vi "GraphAttribute.vi"() -> ()   [LabVIEW 2012, in "WaveGraphX.xctl"]
uses:
  WaveGraphX.xctl
  <resource>/importtools/Common/Event/NISAST Event.lvclass
  GraphStates.ctl
panel:
  in  "曲线条数":u8
  in  "AttrCluster":T1={"曲线条数"=3, "曲线属性簇数组"=[{"曲线_曲线"=0, "曲线_颜色"=16711717, "曲线_线条样式"=0, "曲线_线条宽度"=0, "曲线_直方图"=0, "曲线_插值"=0, "曲线_填充基线"=0, "曲线_点样式"=0}, {"曲线_曲线"=1, "曲线_颜色"=786687, "曲线_线条样式"=1, "曲线_线条宽度"=0, "曲线_直方图"=0, "曲线_插值"=0, "曲线_填充基线"=0, "曲线_点样式"=0}, {"曲线_曲线"=2, "曲线_颜色"=56357, "曲线_线条样式"=2, "曲线_线条宽度"=0, "曲线_直方图"=0, "曲线_插值"=0, "曲线_填充基线"=0, "曲线_点样式"=0}], "文本属性簇数组"=[{"文本_文本"=0, "文本"="标题", "字体"=0, "颜色"=0, "大小"=0, "加粗"=TRUE, "斜体"=FALSE, "下划线"=FALSE}, {"文本_文本"=1, "文本"="", "字体"=0, "颜色"=0, "大小"=0, "加粗"=FALSE, "斜体"=TRUE, "下划线"=FALSE}, {"文本_文本"=2, "文本"="", "字体"=0, "颜色"=0, "大小"=0, "加粗"=FALSE, "斜体"=FALSE, "下划线"=TRUE}, {"文本_文本"=3, "文本"="", "字体"=0, "颜色"=0, "大小"=0, "加粗"=TRUE, "斜体"=TRUE, "下划线"=TRUE}], "信息属性簇"={"图例"=TRUE, "信息_统计量"=FALSE, "信息_统计量_有效值"=TRUE, "信息_统计量_最大值"=TRUE, "信息_统计量_最小值"=FALSE, "信息_统计量_峰峰值"=FALSE, "信息_统计量_均值"=FALSE, "信息_统计量_方差"=FALSE, "信息_统计量_所有通道"=FALSE, "光标列表"=1, "数量"=1.0, "排列"=0, "格式"=0, "精度"=3.0}} {"信息属性簇"."格式" items=["十进制", "科学值"]; "信息属性簇"."排列" items=["幅值"]; "信息属性簇"."光标列表" items=["单光标", "双光标", "峰值光标"]; "曲线属性簇数组"."曲线_填充基线" items=["无", "零", "负无穷大", "正无穷大"]; "曲线属性簇数组"."曲线_线条宽度" items=["0", "1", "2", "3", "4", "5"]; "曲线属性簇数组"."曲线_线条样式" items=["实线", "粗虚线", "细虚线", "点划线", "双点划线"]}
  in  "Event In":refnum<class "NISAST Event.lvclass">
  in  "应用":bool
  in  "取消":bool
  in  "确定":bool
  in  "选项卡控件":enum32{"曲线", "文本", "信息"}(tab)
  in  "曲线_曲线":i32(listbox) caption="曲线"
  in  "曲线_颜色":u32(colorbox) caption="颜色"
  in  "曲线_线条宽度":u16(ring) caption="线条宽度" items=["0", "1", "2", "3", "4", "5"]
  in  "曲线_线条样式":u16(ring) caption="线条样式" items=["实线", "粗虚线", "细虚线", "点划线", "双点划线"]
  in  "曲线_直方图":u16(ring) caption="直方图"
  in  "曲线_插值":u16(ring) caption="插值"
  in  "曲线_填充基线":u16(ring) caption="填充基线" items=["无", "零", "负无穷大", "正无穷大"]
  in  "曲线_点样式":u16(ring) caption="点样式"
  in  "加粗":bool
  in  "大小":u16(ring)
  in  "文本":string
  in  "文本_文本":i32(listbox) caption="文本"
  in  "字体":u16(ring)
  in  "颜色":u16(ring)
  in  "斜体":bool
  in  "下划线":bool
  in  "格式":u16(ring) items=["十进制", "科学值"]
  in  "信息_统计量_所有通道":bool
  in  "信息_统计量":bool
  in  "图例":bool
  in  "信息_统计量_有效值":bool
  in  "信息_统计量_最大值":bool
  in  "信息_统计量_最小值":bool
  in  "信息_统计量_峰峰值":bool
  in  "信息_统计量_均值":bool
  in  "信息_统计量_方差":bool
  in  "光标列表":u16(ring) items=["单光标", "双光标", "峰值光标"]
  in  "数量":dbl=1.0
  in  "排列":u16(ring) items=["幅值"]
  in  "精度":dbl=3.0
  # "光标"
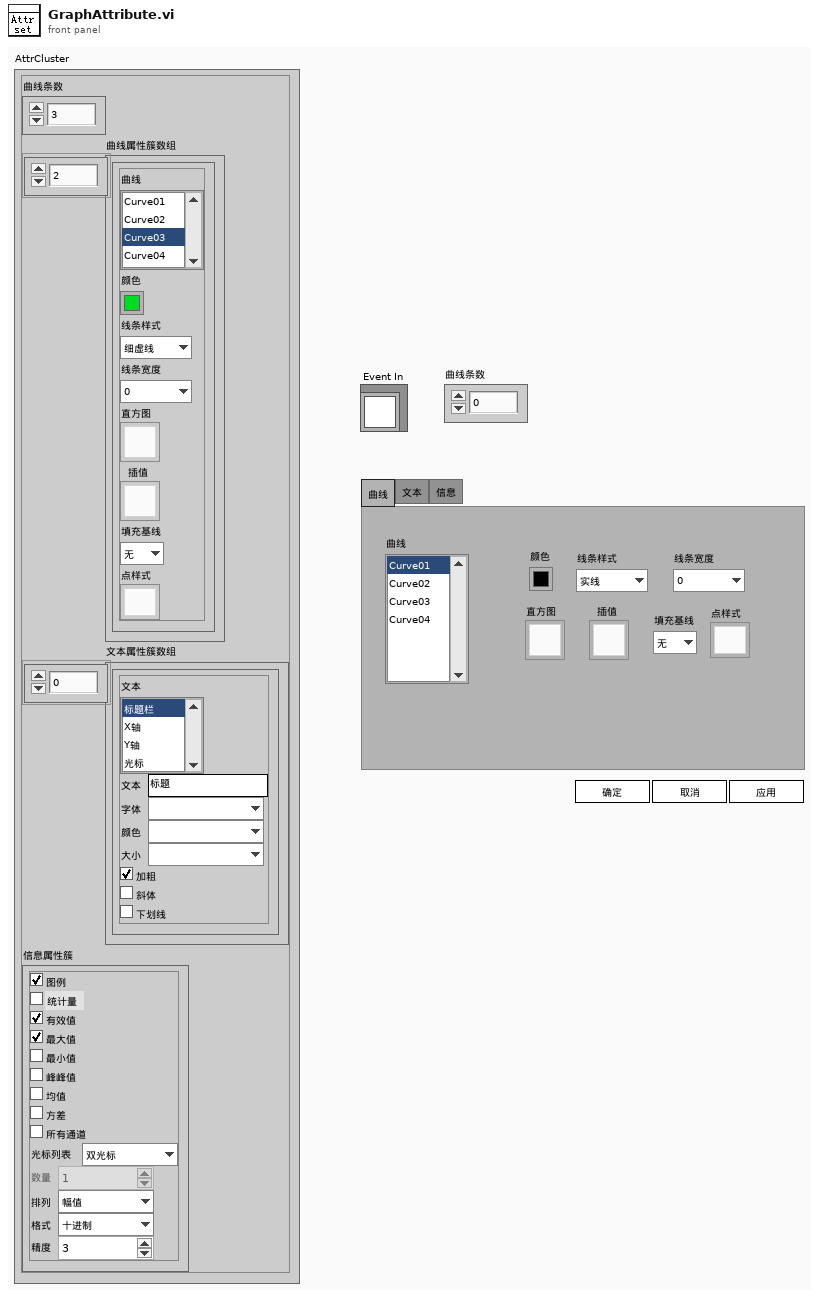
[diagram p1: front panel]
types:
  T1 = typedef "WaveGraphX.xctl/GraphStates.ctl" = cluster{"曲线条数":u8, "曲线属性簇数组":cluster{"曲线_曲线":i32, "曲线_颜色":u32, "曲线_线条样式":u16, "曲线_线条宽度":u16, "曲线_直方图":u16, "曲线_插值":u16, "曲线_填充基线":u16, "曲线_点样式":u16}[], "文本属性簇数组":cluster{"文本_文本":i32, "文本":string, "字体":u16, "颜色":u16, "大小":u16, "加粗":bool, "斜体":bool, "下划线":bool}[], "信息属性簇":cluster{"图例":bool, "信息_统计量":bool, "信息_统计量_有效值":bool, "信息_统计量_最大值":bool, "信息_统计量_最小值":bool, "信息_统计量_峰峰值":bool, "信息_统计量_均值":bool, "信息_统计量_方差":bool, "信息_统计量_所有通道":bool, "光标列表":u16, "数量":dbl, "排列":u16, "格式":u16, "精度":dbl}}
  T2 = cluster{"曲线_曲线":i32, "曲线_颜色":u32, "曲线_线条样式":u16, "曲线_线条宽度":u16, "曲线_直方图":u16, "曲线_插值":u16, "曲线_填充基线":u16, "曲线_点样式":u16}[]
  T3 = cluster{"文本_文本":i32, "文本":string, "字体":u16, "颜色":u16, "大小":u16, "加粗":bool, "斜体":bool, "下划线":bool}[]
  T4 = cluster{"图例":bool, "信息_统计量":bool, "信息_统计量_有效值":bool, "信息_统计量_最大值":bool, "信息_统计量_最小值":bool, "信息_统计量_峰峰值":bool, "信息_统计量_均值":bool, "信息_统计量_方差":bool, "信息_统计量_所有通道":bool, "光标列表":u16, "数量":dbl, "排列":u16, "格式":u16, "精度":dbl}
  T5 = cluster{"曲线_曲线":i32, "曲线_颜色":u32, "曲线_线条样式":u16, "曲线_线条宽度":u16, "曲线_直方图":u16, "曲线_插值":u16, "曲线_填充基线":u16, "曲线_点样式":u16}
  T6 = cluster{"文本_文本":i32, "文本":string, "字体":u16, "颜色":u16, "大小":u16, "加粗":bool, "斜体":bool, "下划线":bool}
  T7 = enum8{"Enabled", "Disabled", "Disabled and Grayed Out"}
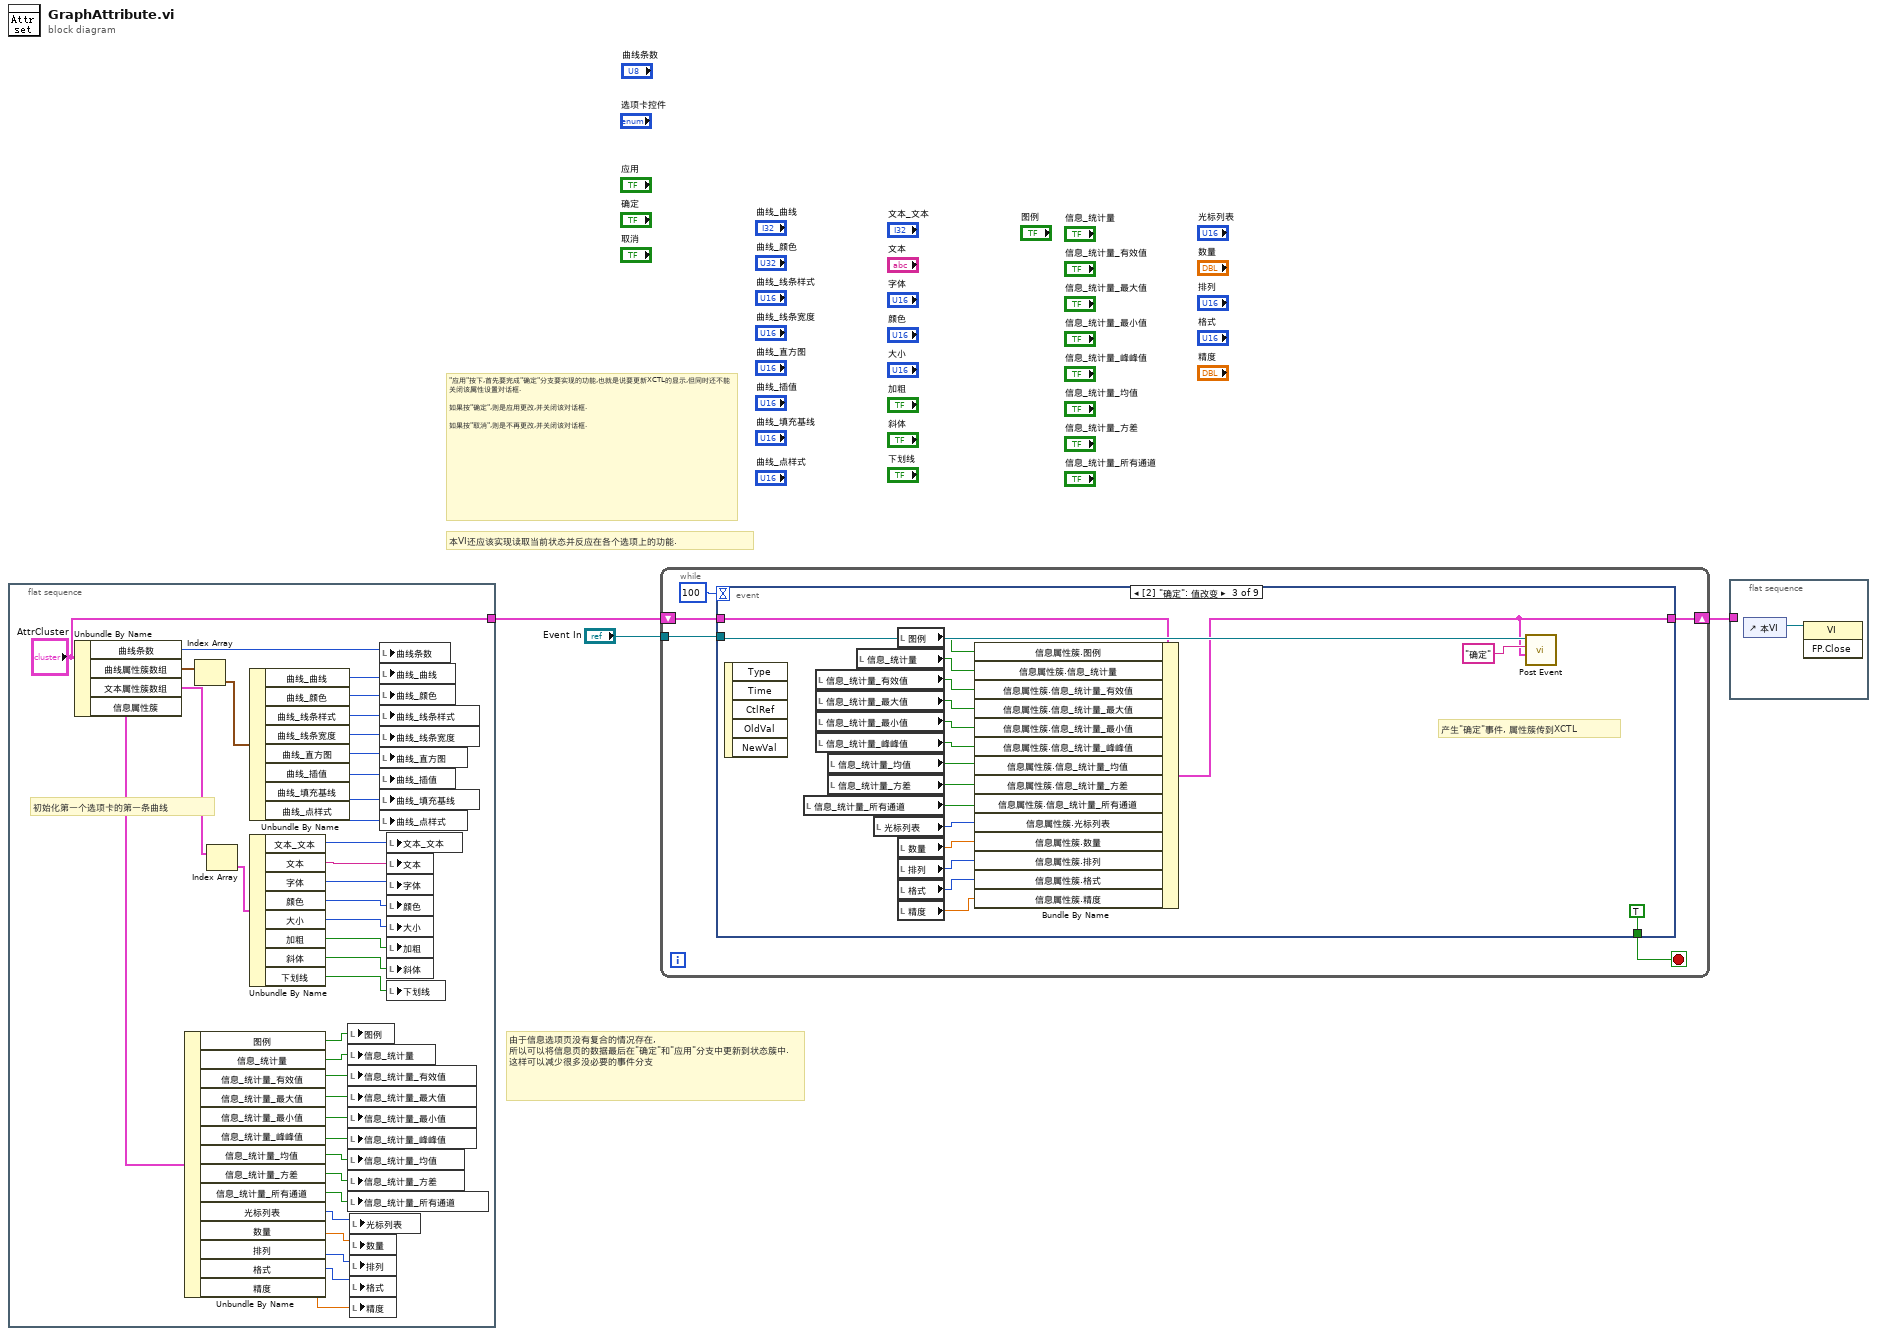
[diagram p0: block diagram]
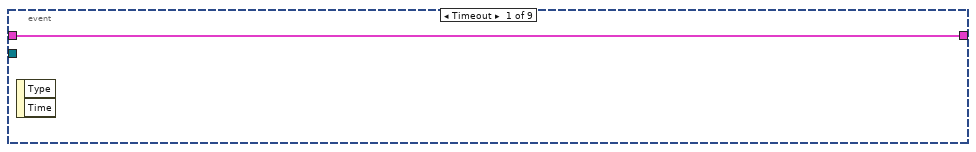
[diagram p2: hidden frame]
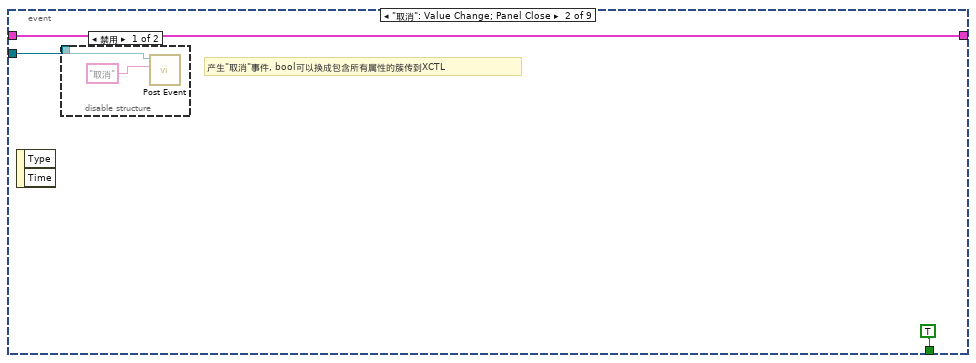
[diagram p3: hidden frame]
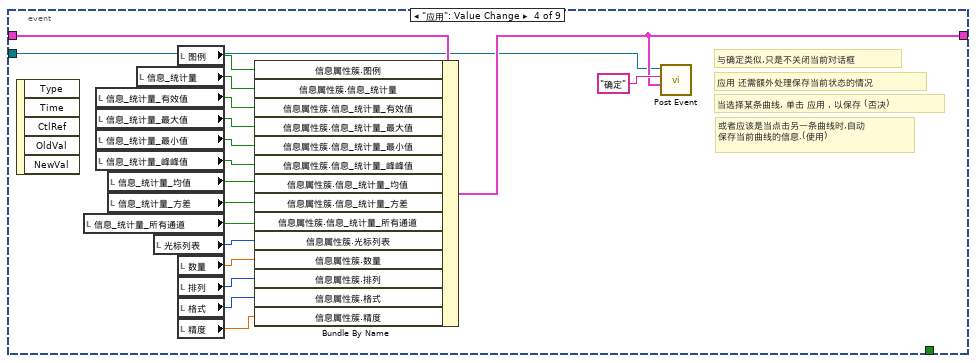
[diagram p5: hidden frame]
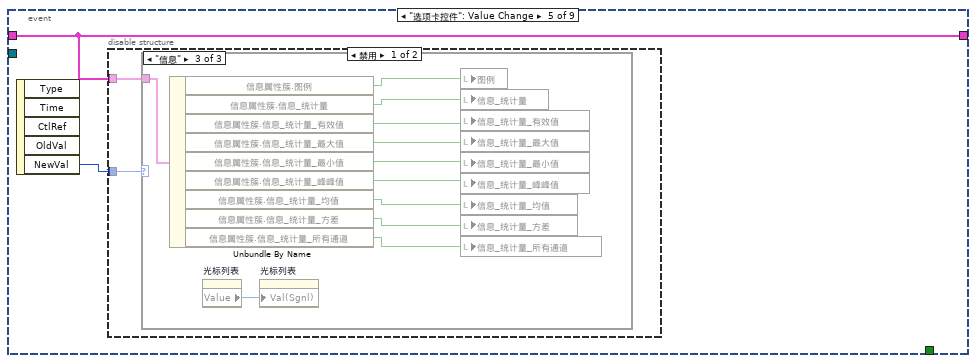
[diagram p6: hidden frame]
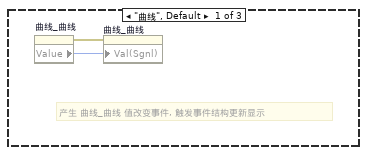
[diagram p7: hidden frame]
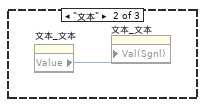
[diagram p8: hidden frame]
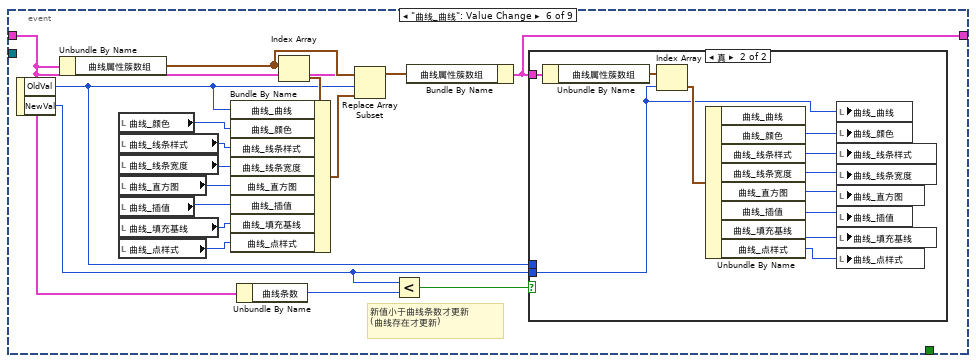
[diagram p10: hidden frame]
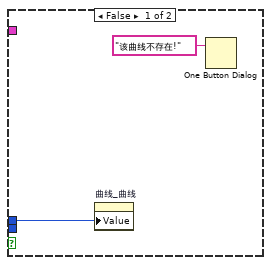
[diagram p11: hidden frame]
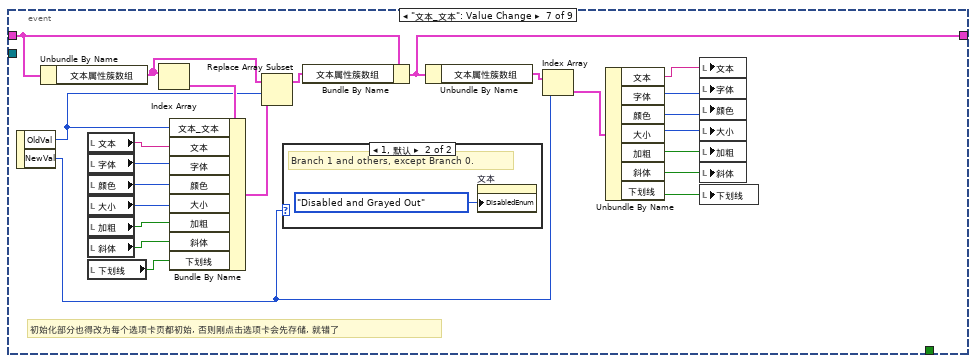
[diagram p12: hidden frame]
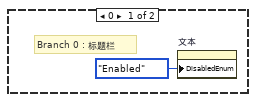
[diagram p13: hidden frame]
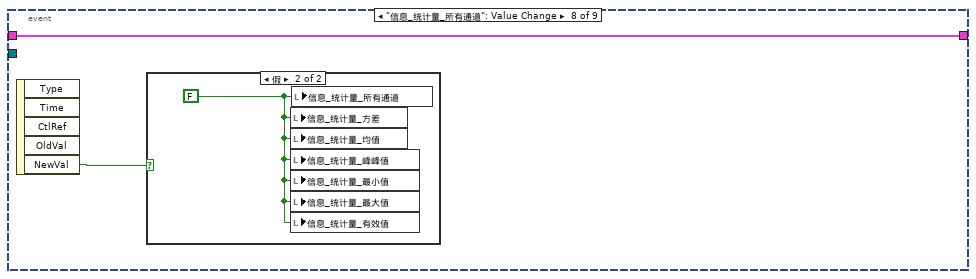
[diagram p14: hidden frame]
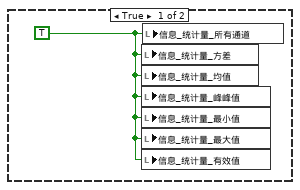
[diagram p15: hidden frame]
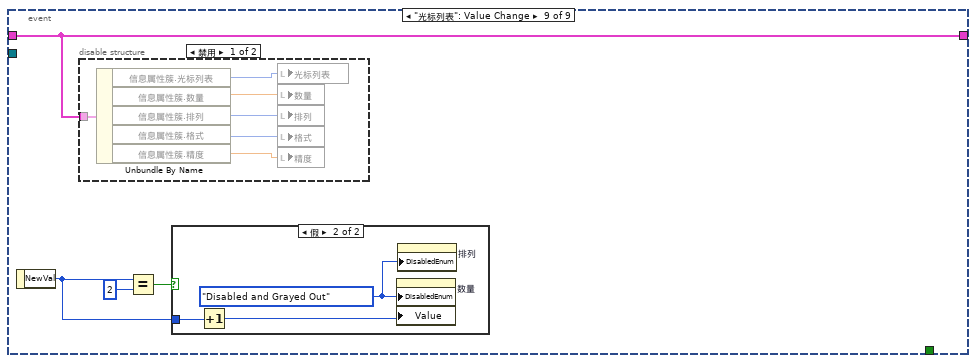
[diagram p16: hidden frame]
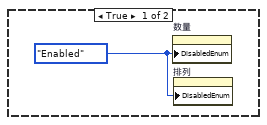
[diagram p18: hidden frame]
diagram:
  # "由于信息选项页没有复合的情况存在, 所以可以将信息页的数据最后在\"确定\"和\"应用\"分支中更新到状态簇中.这样可以减少很多没必要的事件分支"
  # "本VI还应该实现读取当前状态并反应在各个选项上的功能."
  # "\"应用\"按下,首先要完成\"确定\"分支要实现的功能,也就是说要更新XCTL的显示,但同时还不能关闭该属性设置对话框.\n\n如果按\"确定\",则是应用更改,并关闭该对话框.\n\n如果按\"取消\",则是不再更改,并关闭该对话框."
  n1 = flat-sequence {
    tunnel: ["AttrCluster"] -> w2
    frame #0 {
      # "初始化第一个选项卡的第一条曲线"
      n2 = Unbundle By Name("AttrCluster") -> ("曲线条数"=w40:u8, "曲线属性簇数组"=w39:T2, "文本属性簇数组"=w28:T3, "信息属性簇"=w18:T4)
      n3 = Unbundle By Name(w18) -> ("图例"=w10:bool, "信息_统计量"=w9:bool, "信息_统计量_有效值"=w17:bool, "信息_统计量_最大值"=w16:bool, "信息_统计量_最小值"=w15:bool, "信息_统计量_峰峰值"=w14:bool, "信息_统计量_均值"=w13:bool, "信息_统计量_方差"=w12:bool, "信息_统计量_所有通道"=w11:bool, "光标列表"=w8:u16, "数量"=w7:dbl, "排列"=w6:u16, "格式"=w5:u16, "精度"=w4:dbl)
      n4 = Index Array(array=w39) -> (element=w38:T5)  [unwired: 1 in]
      n5 = Index Array(array=w28) -> (element=w27:T6)  [unwired: 1 in]
      n6 = Unbundle By Name(w38) -> ("曲线_曲线"=w37:i32, "曲线_颜色"=w36:u32, "曲线_线条样式"=w35:u16, "曲线_线条宽度"=w34:u16, "曲线_直方图"=w33:u16, "曲线_插值"=w32:u16, "曲线_填充基线"=w31:u16, "曲线_点样式"=w30:u16)
      n7 = Unbundle By Name(w27) -> ("文本_文本"=w19:i32, "文本"=w26:string, "字体"=w25:u16, "颜色"=w24:u16, "大小"=w23:u16, "加粗"=w22:bool, "斜体"=w21:bool, "下划线"=w20:bool)
      n8 = local write "图例"(w10) -> ()
      n9 = local write "信息_统计量"(w9) -> ()
      n10 = local write "信息_统计量_有效值"(w17) -> ()
      n11 = local write "信息_统计量_最大值"(w16) -> ()
      n12 = local write "信息_统计量_最小值"(w15) -> ()
      n13 = local write "信息_统计量_峰峰值"(w14) -> ()
      n14 = local write "信息_统计量_均值"(w13) -> ()
      n15 = local write "信息_统计量_方差"(w12) -> ()
      n16 = local write "信息_统计量_所有通道"(w11) -> ()
      n17 = local write "光标列表"(w8) -> ()
      n18 = local write "数量"(w7) -> ()
      n19 = local write "排列"(w6) -> ()
      n20 = local write "格式"(w5) -> ()
      n21 = local write "精度"(w4) -> ()
      n22 = local write "曲线条数"(w40) -> ()
      n23 = local write "曲线_曲线"(w37) -> ()
      n24 = local write "曲线_颜色"(w36) -> ()
      n25 = local write "曲线_线条样式"(w35) -> ()
      n26 = local write "曲线_线条宽度"(w34) -> ()
      n27 = local write "曲线_直方图"(w33) -> ()
      n28 = local write "曲线_插值"(w32) -> ()
      n29 = local write "曲线_填充基线"(w31) -> ()
      n30 = local write "曲线_点样式"(w30) -> ()
      n31 = local write "文本_文本"(w19) -> ()
      n32 = local write "文本"(w26) -> ()
      n33 = local write "字体"(w25) -> ()
      n34 = local write "颜色"(w24) -> ()
      n35 = local write "大小"(w23) -> ()
      n36 = local write "加粗"(w22) -> ()
      n37 = local write "斜体"(w21) -> ()
      n38 = local write "下划线"(w20) -> ()
    }
  }
  n39 = while {
    tunnel: "Event In" -> [w44]
    shift-right: [w41] -> w1
    shift-left: w2 -> [w42]
    stop <- w45 stop-if-true
    n40 = event shown="[2] \"确定\": 值改变" {
      selector: _ -> [_ _ _ _ _ _ _ _ _]
      dyn-events: _ -> [_ _ _ _ _ _ _ _ _]
      timeout: 100 -> [_ _ _ _ _ _ _ _ _]
      tunnel: [_ TRUE TRUE _ _ _ _ _ _] -> w45
      tunnel: w44 -> [_ w48 w69 w71 _ _ _ _ _]
      tunnel: w42 -> [w46 w47 w53 w88 w89 w110 w148 w163 w167]
      tunnel: [w46 w47 w52 w72 w89 w112 w147 w163 w167] -> w41
      event Timeout {
        n41 = event-data() -> ()  [unwired: 1 in, 2 out]
      }
      event "取消": Value Change; Panel Close {
        # "产生\"取消\"事件, bool可以换成包含所有属性的簇传到XCTL"
        n42 = event-data() -> ()  [unwired: 1 in, 2 out]
        n43 = disable-structure shown="禁用" {
          disable-tunnel: w48 -> [w50 _]
          frame Disabled {
            n44 = call-dynamic "Post Event.vi"("Event Name"="取消", "Event in"=w50) -> ()  [unwired: 8 in, 2 out]
          }
          frame Enabled {
          }
        }
      }
      event "确定": Value Change {
        # "产生\"确定\"事件, 属性簇传到XCTL"
        n45 = event-data() -> ()  [unwired: 1 in, 5 out]
        n46 = local read "信息_统计量_所有通道"() -> (w59:bool)
        n47 = local read "信息_统计量_有效值"() -> (w65:bool)
        n48 = local read "信息_统计量_最大值"() -> (w64:bool)
        n49 = local read "信息_统计量_最小值"() -> (w63:bool)
        n50 = local read "信息_统计量_峰峰值"() -> (w62:bool)
        n51 = local read "信息_统计量_均值"() -> (w61:bool)
        n52 = local read "信息_统计量_方差"() -> (w60:bool)
        n53 = local read "信息_统计量"() -> (w66:bool)
        n54 = local read "光标列表"() -> (w58:u16)
        n55 = local read "图例"() -> (w67:bool)
        n56 = local read "数量"() -> (w57:dbl)
        n57 = local read "排列"() -> (w56:u16)
        n58 = local read "格式"() -> (w55:u16)
        n59 = local read "精度"() -> (w54:dbl)
        n60 = Bundle By Name(cluster=w53, "信息属性簇.图例"=w67, "信息属性簇.信息_统计量"=w66, "信息属性簇.信息_统计量_有效值"=w65, "信息属性簇.信息_统计量_最大值"=w64, "信息属性簇.信息_统计量_最小值"=w63, "信息属性簇.信息_统计量_峰峰值"=w62, "信息属性簇.信息_统计量_均值"=w61, "信息属性簇.信息_统计量_方差"=w60, "信息属性簇.信息_统计量_所有通道"=w59, "信息属性簇.光标列表"=w58, "信息属性簇.数量"=w57, "信息属性簇.排列"=w56, "信息属性簇.格式"=w55, "信息属性簇.精度"=w54) -> (w52:T1)
        n61 = call-dynamic "Post Event.vi"("Event Data"=w52, "Event Name"="确定", "Event in"=w69) -> ()  [unwired: 7 in, 2 out]
      }
      event "应用": Value Change {
        # "或者应该是当点击另一条曲线时,自动\n保存当前曲线的信息.(使用)"
        # "当选择某条曲线, 单击 应用 , 以保存 (否决)"
        # "应用 还需额外处理保存当前状态的情况"
        # "与确定类似,只是不关闭当前对话框"
        n62 = event-data() -> ()  [unwired: 1 in, 5 out]
        n63 = local read "信息_统计量_所有通道"() -> (w79:bool)
        n64 = local read "信息_统计量_有效值"() -> (w85:bool)
        n65 = local read "信息_统计量_最大值"() -> (w84:bool)
        n66 = local read "信息_统计量_最小值"() -> (w83:bool)
        n67 = local read "信息_统计量_峰峰值"() -> (w82:bool)
        n68 = local read "信息_统计量_均值"() -> (w81:bool)
        n69 = local read "信息_统计量_方差"() -> (w80:bool)
        n70 = local read "信息_统计量"() -> (w86:bool)
        n71 = local read "光标列表"() -> (w78:u16)
        n72 = local read "图例"() -> (w87:bool)
        n73 = local read "数量"() -> (w77:dbl)
        n74 = local read "排列"() -> (w76:u16)
        n75 = local read "格式"() -> (w75:u16)
        n76 = local read "精度"() -> (w74:dbl)
        n77 = Bundle By Name(cluster=w88, "信息属性簇.图例"=w87, "信息属性簇.信息_统计量"=w86, "信息属性簇.信息_统计量_有效值"=w85, "信息属性簇.信息_统计量_最大值"=w84, "信息属性簇.信息_统计量_最小值"=w83, "信息属性簇.信息_统计量_峰峰值"=w82, "信息属性簇.信息_统计量_均值"=w81, "信息属性簇.信息_统计量_方差"=w80, "信息属性簇.信息_统计量_所有通道"=w79, "信息属性簇.光标列表"=w78, "信息属性簇.数量"=w77, "信息属性簇.排列"=w76, "信息属性簇.格式"=w75, "信息属性簇.精度"=w74) -> (w72:T1)
        n78 = call-dynamic "Post Event.vi"("Event Data"=w72, "Event Name"="确定", "Event in"=w71) -> ()  [unwired: 7 in, 2 out]
      }
      event "选项卡控件": Value Change {
        n79 = event-data() -> ("NewVal"=w90:enum32{"曲线", "文本", "信息"})  [unwired: 1 in, 4 out]
        n80 = disable-structure shown="禁用" {
          disable-tunnel: w90 -> [w92 _]
          disable-tunnel: w89 -> [w91 _]
          frame Disabled {
            n81 = case shown="\"信息\"" w92 {
              tunnel: w91 -> [_ _ w106]
              frame "曲线", Default {
                # "产生 曲线_曲线 值改变事件, 触发事件结构更新显示"
                n82 = property on="曲线_曲线" class="LstBox (严格)"() -> (error out=w94:errorcluster, "Value"=w93:i32)  [unwired: 2 in, 1 out]
                n83 = property on="曲线_曲线" class="LstBox (严格)"(error in=w94, "Val(Sgnl)"=w93) -> ()  [unwired: 1 in, 2 out]
              }
              frame "文本" {
                n84 = property on="文本_文本" class="LstBox (严格)"() -> ("Value"=w95:i32)  [unwired: 2 in, 2 out]
                n85 = property on="文本_文本" class="LstBox (严格)"("Val(Sgnl)"=w95) -> ()  [unwired: 2 in, 2 out]
              }
              frame "信息" {
                n86 = Unbundle By Name(w106) -> ("信息属性簇.图例"=w105:bool, "信息属性簇.信息_统计量"=w104:bool, "信息属性簇.信息_统计量_有效值"=w103:bool, "信息属性簇.信息_统计量_最大值"=w102:bool, "信息属性簇.信息_统计量_最小值"=w101:bool, "信息属性簇.信息_统计量_峰峰值"=w100:bool, "信息属性簇.信息_统计量_均值"=w99:bool, "信息属性簇.信息_统计量_方差"=w98:bool, "信息属性簇.信息_统计量_所有通道"=w97:bool)
                n87 = property on="光标列表" class="Ring (严格)"() -> ("Value"=w96:u16)  [unwired: 2 in, 2 out]
                n88 = property on="光标列表" class="Ring (严格)"("Val(Sgnl)"=w96) -> ()  [unwired: 2 in, 2 out]
                n89 = local write "图例"(w105) -> ()
                n90 = local write "信息_统计量"(w104) -> ()
                n91 = local write "信息_统计量_有效值"(w103) -> ()
                n92 = local write "信息_统计量_最大值"(w102) -> ()
                n93 = local write "信息_统计量_最小值"(w101) -> ()
                n94 = local write "信息_统计量_峰峰值"(w100) -> ()
                n95 = local write "信息_统计量_均值"(w99) -> ()
                n96 = local write "信息_统计量_方差"(w98) -> ()
                n97 = local write "信息_统计量_所有通道"(w97) -> ()
              }
            }
          }
          frame Enabled {
          }
        }
      }
      event "曲线_曲线": Value Change {
        # "新值小于曲线条数才更新\n(曲线存在才更新)"
        n98 = event-data() -> ("OldVal"=w107:i32, "NewVal"=w111:i32)  [unwired: 1 in]
        n99 = Unbundle By Name(w110) -> ("曲线属性簇数组"=w114:T2)
        n100 = local read "曲线_颜色"() -> (w123:u32)
        n101 = local read "曲线_线条样式"() -> (w122:u16)
        n102 = local read "曲线_线条宽度"() -> (w121:u16)
        n103 = local read "曲线_直方图"() -> (w120:u16)
        n104 = local read "曲线_插值"() -> (w119:u16)
        n105 = local read "曲线_填充基线"() -> (w118:u16)
        n106 = local read "曲线_点样式"() -> (w117:u16)
        n107 = Unbundle By Name(w110) -> ("曲线条数"=w109:u8)
        n108 = Index Array(array=w114) -> (element=w116:T5)  [unwired: 1 in]
        n109 = Bundle By Name(cluster=w116, "曲线_曲线"=w107, "曲线_颜色"=w123, "曲线_线条样式"=w122, "曲线_线条宽度"=w121, "曲线_直方图"=w120, "曲线_插值"=w119, "曲线_填充基线"=w118, "曲线_点样式"=w117) -> (w115:T5)
        n110 = Replace Array Subset(array=w114, new element=w115, index=w107) -> (w113:T2)
        n111 = Less?(x=w111, y=w109) -> (x < y?=w108:bool)
        n112 = Bundle By Name(cluster=w110, "曲线属性簇数组"=w113) -> (w112:T1)
        n113 = case shown="真" w108 {
          tunnel: w112 -> [_ w129]
          tunnel: w111 -> [_ w126]
          tunnel: w107 -> [w124 _]
          frame False {
            n114 = property on="曲线_曲线" class="LstBox (严格)"("Value"=w124) -> ()  [unwired: 2 in, 2 out]
            n115 = One Button Dialog(message="该曲线不存在!" ("消息")) -> ()  [unwired: 1 in, 1 out]
          }
          frame True {
            n116 = Unbundle By Name(w129) -> ("曲线属性簇数组"=w128:T2)
            n117 = Index Array(array=w128, index=w126) -> (element=w127:T5)
            n118 = Unbundle By Name(w127) -> ("曲线_颜色"=w130:u32, "曲线_线条样式"=w131:u16, "曲线_线条宽度"=w132:u16, "曲线_直方图"=w133:u16, "曲线_插值"=w134:u16, "曲线_填充基线"=w135:u16, "曲线_点样式"=w136:u16)  [unwired: 1 out]
            n119 = local write "曲线_曲线"(w126) -> ()
            n120 = local write "曲线_颜色"(w130) -> ()
            n121 = local write "曲线_线条样式"(w131) -> ()
            n122 = local write "曲线_线条宽度"(w132) -> ()
            n123 = local write "曲线_直方图"(w133) -> ()
            n124 = local write "曲线_插值"(w134) -> ()
            n125 = local write "曲线_填充基线"(w135) -> ()
            n126 = local write "曲线_点样式"(w136) -> ()
          }
        }
      }
      event "文本_文本": Value Change {
        # "初始化部分也得改为每个选项卡页都初始, 否则刚点击选项卡会先存储, 就错了"
        n127 = event-data() -> ("OldVal"=w150:i32, "NewVal"=w145:i32)  [unwired: 1 in]
        n128 = Unbundle By Name(w148) -> ("文本属性簇数组"=w149:T3)
        n129 = local read "文本"() -> (w159:string)
        n130 = local read "字体"() -> (w158:u16)
        n131 = local read "颜色"() -> (w157:u16)
        n132 = local read "大小"() -> (w156:u16)
        n133 = local read "加粗"() -> (w155:bool)
        n134 = local read "斜体"() -> (w154:bool)
        n135 = local read "下划线"() -> (w153:bool)
        n136 = Index Array(array=w149) -> (element=w160:T6)  [unwired: 1 in]
        n137 = Bundle By Name(cluster=w160, "文本_文本"=w150, "文本"=w159, "字体"=w158, "颜色"=w157, "大小"=w156, "加粗"=w155, "斜体"=w154, "下划线"=w153) -> (w151:T6)
        n138 = Replace Array Subset(array=w149, new element=w151, index=w150) -> (w152:T3)
        n139 = case shown="1, 默认" w145 {
          frame 0 {
            # "Branch 0 : 标题栏"
            n140 = property on="文本" class="Str"("DisabledEnum"=T7."Enabled" ("禁用")) -> ()  [unwired: 2 in, 2 out]
          }
          frame 1, Default {
            # "Branch 1 and others, except Branch 0."
            n141 = property on="文本" class="Str"("DisabledEnum"=T7."Disabled and Grayed Out" ("禁用")) -> ()  [unwired: 2 in, 2 out]
          }
        }
        n142 = Bundle By Name(cluster=w148, "文本属性簇数组"=w152) -> (w147:T1)
        n143 = Unbundle By Name(w147) -> ("文本属性簇数组"=w146:T3)
        n144 = Index Array(array=w146, index=w145) -> (element=w137:T6)
        n145 = Unbundle By Name(w137) -> ("文本"=w144:string, "字体"=w143:u16, "颜色"=w142:u16, "大小"=w141:u16, "加粗"=w140:bool, "斜体"=w139:bool, "下划线"=w138:bool)
        n146 = local write "文本"(w144) -> ()
        n147 = local write "字体"(w143) -> ()
        n148 = local write "颜色"(w142) -> ()
        n149 = local write "大小"(w141) -> ()
        n150 = local write "加粗"(w140) -> ()
        n151 = local write "斜体"(w139) -> ()
        n152 = local write "下划线"(w138) -> ()
      }
      event "信息_统计量_所有通道": Value Change {
        n153 = event-data() -> ("NewVal"=w164:bool)  [unwired: 1 in, 4 out]
        n154 = case shown="假" w164 {
          frame True {
            w165 = TRUE ("信息_统计量_所有通道")
            n155 = local write "信息_统计量_方差"(w165) -> ()
            n156 = local write "信息_统计量_均值"(w165) -> ()
            n157 = local write "信息_统计量_峰峰值"(w165) -> ()
            n158 = local write "信息_统计量_最小值"(w165) -> ()
            n159 = local write "信息_统计量_最大值"(w165) -> ()
            n160 = local write "信息_统计量_有效值"(w165) -> ()
            n161 = local write "信息_统计量_所有通道"(w165) -> ()
          }
          frame False {
            w166 = FALSE ("信息_统计量_所有通道")
            n162 = local write "信息_统计量_方差"(w166) -> ()
            n163 = local write "信息_统计量_均值"(w166) -> ()
            n164 = local write "信息_统计量_峰峰值"(w166) -> ()
            n165 = local write "信息_统计量_最小值"(w166) -> ()
            n166 = local write "信息_统计量_最大值"(w166) -> ()
            n167 = local write "信息_统计量_有效值"(w166) -> ()
            n168 = local write "信息_统计量_所有通道"(w166) -> ()
          }
        }
      }
      event "光标列表": Value Change {
        n169 = event-data() -> ("NewVal"=w168:u16)  [unwired: 1 in]
        n170 = disable-structure shown="禁用" {
          disable-tunnel: w167 -> [w171 _]
          frame Disabled {
            n171 = Unbundle By Name(w171) -> ("信息属性簇.光标列表"=w172:u16, "信息属性簇.数量"=w173:dbl, "信息属性簇.排列"=w176:u16, "信息属性簇.格式"=w175:u16, "信息属性簇.精度"=w174:dbl)
            n172 = local write "光标列表"(w172) -> ()
            n173 = local write "数量"(w173) -> ()
            n174 = local write "排列"(w176) -> ()
            n175 = local write "格式"(w175) -> ()
            n176 = local write "精度"(w174) -> ()
          }
          frame Enabled {
          }
        }
        n177 = Equal?(x=w168, y=u16 2) -> (x = y?=w169:bool)
        n178 = case shown="假" w169 {
          tunnel: w168 -> [_ w180]
          frame True {
            w177 = T7."Enabled" ("禁用")
            n179 = property on="数量" class="DigNum (严格)"("DisabledEnum"=w177) -> ()  [unwired: 2 in, 2 out]
            n180 = property on="排列" class="Ring (严格)"("DisabledEnum"=w177) -> ()  [unwired: 2 in, 2 out]
          }
          frame False {
            w178 = T7."Disabled and Grayed Out" ("禁用")
            n181 = Increment(x=w180) -> (x+1=w179:u16)
            n182 = property on="数量" class="DigNum (严格)"("DisabledEnum"=w178, "Value"=w179) -> ()  [unwired: 2 in, 2 out]
            n183 = property on="排列" class="Ring (严格)"("DisabledEnum"=w178) -> ()  [unwired: 2 in, 2 out]
          }
        }
      }
    }
  }
  n184 = flat-sequence {
    tunnel: w1 -> [_]
    frame #0 {
      n185 = control-ref of="本VI"() -> (w181:refnum<vi>)
      n186 = invoke class="VI" method="FP.Close"(reference=w181) -> ()  [unwired: 2 in, 3 out]
    }
  }
